vi "Autosize Table Columns.vi"(8 "error in (no error)":errorcluster, 9 "Resize Table?":bool, 10 "Table Ref":refnum<vi>, 11 "State":T1={"logTable"=refnum, "max items"=500, "displaydata"=[], "data"=[], "Auto Scroll"=TRUE, "current item"=500, "col headers"=[], "Add to Top"=TRUE, "Auto resize"=TRUE, "col size"=[], "filters"=[], "color cells"=[]}) -> (0 "error out":errorcluster, 2 "Table Ref (dup)":refnum<vi>, 3 "State (dup)":T1={"logTable"=refnum, "max items"=500, "displaydata"=[], "data"=[], "Auto Scroll"=TRUE, "current item"=500, "col headers"=[], "Add to Top"=TRUE, "Auto resize"=TRUE, "col size"=[], "filters"=[], "color cells"=[]})   [LabVIEW 2014, in "UI-DisplayTable(dev).xctl"]
doc: "This VI resizes each column of the table specified by Table Ref based on the widest entry of the column. Additionally, if Resize Table? is TRUE, the VI will set the table width based on the number of populated columns."
uses:
  UI-DisplayTable(dev).xctl
  State.ctl
  DEF-Filter.ctl
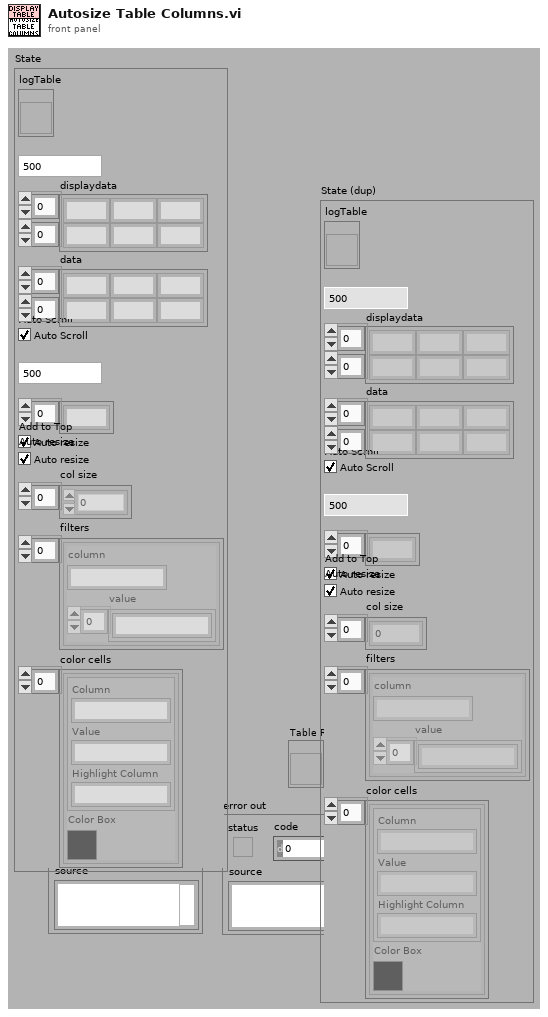
[diagram p1: front panel]
types:
  T1 = typedef "UI-DisplayTable(dev).xctl/State.ctl" = cluster{"logTable":refnum<vi>, "max items":i32, "displaydata":string[][], "data":string[][], "Auto Scroll":bool, "current item":i32, "col headers":string[], "Add to Top":bool, "Auto resize":bool, "col size":i32[], "filters":T2[], "color cells":cluster{"color cell":cluster{"Column":string, "Value":string, "Highlight Column":string}, "Color Box":u32}[]}
  T2 = typedef "UI-DisplayTable(dev).xctl/DEF-Filter.ctl" = cluster{"column":string, "value":string[]}
  T3 = enum16{"User-specified Font", "Application Font", "System Font", "Dialog Font"}
  T4 = cluster{"Font Name:":string, "Size":i16, "Strikeout?":bool, "Italic?":bool, "Underline?":bool, "Outline?":bool, "Shadow?":bool, "Bold?":bool}
  T5 = cluster{"left":i16, "top":i16, "right":i16, "bottom":i16}
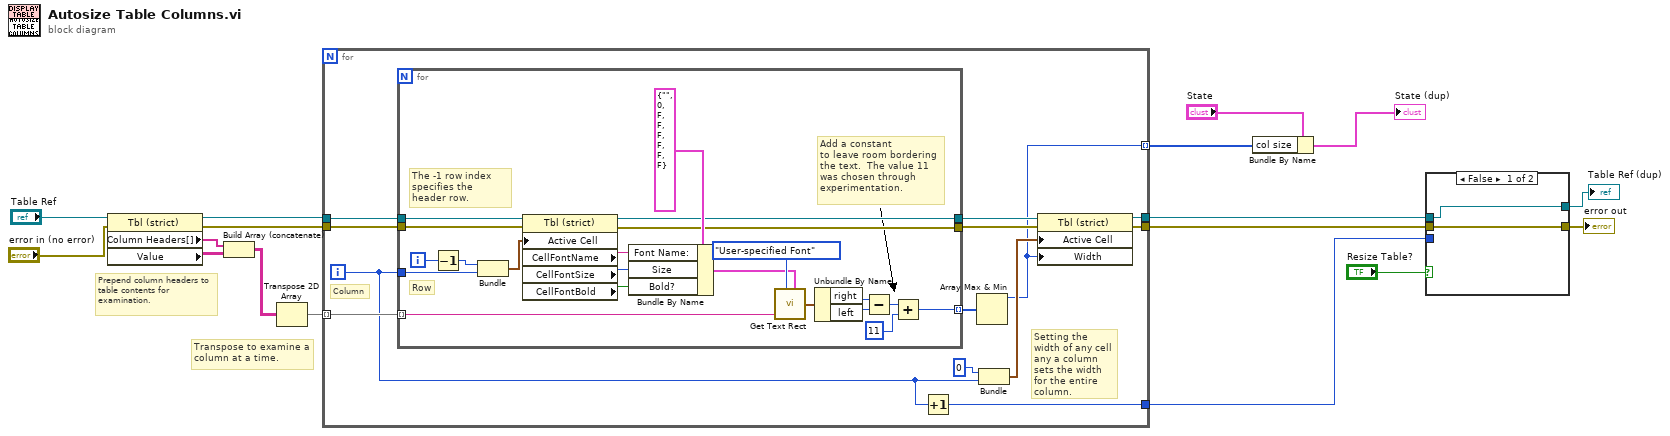
[diagram p0: block diagram]
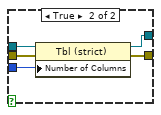
[diagram p2: hidden frame]
diagram:
  # "Transpose to examine a column at a time."
  # "Prepend column headers to table contents for examination."
  n1 = property class="Tbl (strict)"(reference="Table Ref", error in="error in (no error)") -> (reference out=w17:refnum<vi>, error out=w13:errorcluster, "Column Headers[]"=w16:string[], "Value"=w12:string[][])
  n2 = Build Array (concatenate)(w16, w12) -> (w15:string[][])
  n3 = Transpose 2D Array(2D array=w15) -> (transposed array=w14:string[][])
  n4 = for {
    tunnel: w14 -> [w30] mode=indexing
    tunnel: w17 -> [w29]
    tunnel: w13 -> [w27]
    tunnel: [w22] -> w7
    tunnel: [w21] -> w8
    tunnel: [w19] -> w6
    tunnel: [w18] -> w1 mode=indexing
    i -> [w20]
    # "Setting the width of any cell any a column sets the width for the entire column."
    # "Column"
    n5 = for {
      tunnel: w30 -> [w43] mode=indexing
      tunnel: w29 -> [w51]
      tunnel: w20 -> [w50]
      tunnel: [w32] -> w28 mode=indexing
      tunnel: w27 -> [w37]
      tunnel: [w36] -> w25
      tunnel: [w35] -> w26
      i -> [w39]
      # "The -1 row index specifies the header row."
      # "Add a constant\nto leave room bordering the text.  The value 11 was chosen through experimentation."
      # "Row"
      n6 = Decrement(x=w39) -> (x-1=w38:i32)
      n7 = Bundle(w38, w50) -> (w49:cluster{i32, i32})  [unwired: 1 in]
      n8 = property class="Tbl (strict)"(reference=w51, error in=w37, "Active Cell"=w49) -> (reference out=w35:refnum<vi>, error out=w36:errorcluster, "CellFontName"=w47:string, "CellFontSize"=w33:u32, "CellFontBold"=w46:bool)
      n9 = Bundle By Name(cluster=T4 {"Font Name:"="", "Size"=0, "Strikeout?"=FALSE, "Italic?"=FALSE, "Underline?"=FALSE, "Outline?"=FALSE, "Shadow?"=FALSE, "Bold?"=FALSE} ("[user-specified font]"), "Font Name:"=w47, "Size"=w33, "Bold?"=w46) -> (w44:T4)
      n10 = call <vilib>:"Get Text Rect.vi"("desired font(Application)"=T3."User-specified Font", "text"=w43, "[user-specified font]"=w44) -> ("rect"=w42:T5)  [unwired: 6 in]
      n11 = Unbundle By Name(w42) -> ("right"=w41:i16, "left"=w40:i16)
      n12 = Subtract(x=w41, y=w40) -> (x-y=w34:i16)
      n13 = Add(x=w34, y=i16 11) -> (x+y=w32:i16)
    }
    n14 = Increment(x=w20) -> (x+1=w19:i32)
    n15 = Array Max & Min(array=w28) -> (max value=w18:i16)  [unwired: 3 out]
    n16 = Bundle(0, w20) -> (w23:cluster{i32, i32})  [unwired: 1 in]
    n17 = property class="Tbl (strict)"(reference=w26, error in=w25, "Active Cell"=w23, "Width"=w18) -> (reference out=w21:refnum<vi>, error out=w22:errorcluster)
  }
  n18 = Bundle By Name(cluster="State", "col size"=w1) -> (→"State (dup)":T1)
  n19 = case shown="False" "Resize Table?" {
    tunnel: w8 -> [w52 w58]
    tunnel: w7 -> [w53 w57]
    tunnel: w6 -> [_ w56]
    tunnel: [w53 w55] -> w5
    tunnel: [w52 w54] -> w4
    frame False {
    }
    frame True {
      n20 = property class="Tbl (strict)"(reference=w58, error in=w57, "Number of Columns"=w56) -> (reference out=w54:refnum<vi>, error out=w55:errorcluster)
    }
  }
  "error out" <- w5
  "Table Ref (dup)" <- w4
